vi "templates CUSTOMFID data keys.vi"(9 "Template Keys":T1, 10 "HTM Keys":T1) -> (2 "HTM Keys":T1)   [LabVIEW 2011]
uses:
  Addons/internet/utils/keyedarr.llb/Keyed Array.ctl
  Addons/internet/utils/strutil.llb/Case Matching.ctl
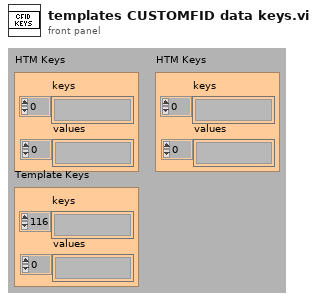
[diagram p1: front panel]
types:
  T1 = typedef "Keyed Array.ctl" = cluster{"keys":string[], "values":string[]}
  T2 = typedef "Case Matching.ctl" = enum16{"a != A", "a == A", "system"}
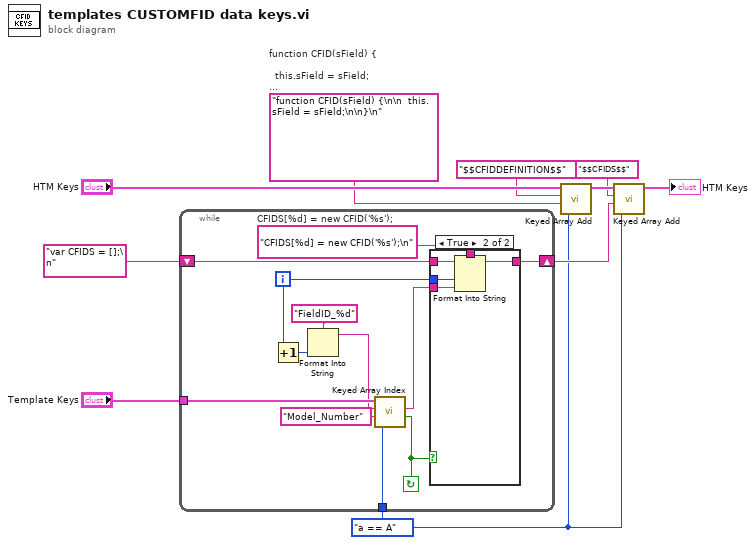
[diagram p0: block diagram]
diagram:
  w2 = Case_Matching."a == A" ("case matching (sensitive)")
  w7 = "function CFID(sField) {\n\n  this.sField = sField;\n\n}\n"  # function CFID(sField) {    this.sField = sField;  }
  n1 = while {
    shift-right: [w20] -> w4
    shift-left: "var CFIDS = [];\n" ("format string") -> [w21]
    tunnel: "Template Keys" -> [w16]
    tunnel: w2 -> [w12]
    i -> [w15]
    stop <- w13 continue-if-true
    w22 = "CFIDS[%d] = new CFID('%s');\n"  # CFIDS[%d] = new CFID('%s');
    n2 = Increment(x=w15) -> (x+1=w14:i32)
    n3 = Format Into String(format string="FieldID_%d", w14) -> (resulting string=w11:string)  [unwired: 2 in, 1 out]
    n4 = call "Keyed Array Index.vi"("case matching (sensitive)"=w12, "default value"="Model_Number", "key"=w11, "array in"=w16) -> ("valid key"=w13:bool, "value"=w17:string)  [unwired: 2 out]
    n5 = case shown="True" w13 {
      tunnel: w22 -> [_ w28]
      tunnel: w21 -> [w23 w27]
      tunnel: [w23 w26] -> w20
      tunnel: w17 -> [_ w25]
      tunnel: w15 -> [_ w24]
      frame False {
      }
      frame True {
        n6 = Format Into String(format string=w28, initial string=w27, w24, w25) -> (resulting string=w26:string)  [unwired: 1 in, 1 out]
      }
    }
  }
  n7 = call "Keyed Array Add.vi"("case matching (sensitive)"=w2, "value"=w7, "key"="$$CFIDDEFINITION$$", "array in"="HTM Keys") -> ("array out"=w6:T1)  [unwired: 3 out]
  n8 = call "Keyed Array Add.vi"("case matching (sensitive)"=w2, "value"=w4, "key"="$$CFIDS$$", "array in"=w6) -> ("array out"=→"HTM Keys":T1)  [unwired: 3 out]
